vi "Configure Glitch Trigger Source.vi"(0 "VISA Resource Name":refnum<visa-resource-name>, 1 "Glitch Polarity (Positive)":i32(slide), 5 "Trigger Source (Channel 1)":string(combo)="CH1", 7 "Trigger Level (0.0 V)":dbl format="%.2p", 9 "Glitch Width (10.0e-6 s)":dbl=1e-05 format="%.2p", 11 "error in (no error)":errorcluster {"code" format="%.0x"}, 12 "Glitch Condition (Less Than)":string(combo)="Less Than") -> (4 "VISA Resource Name Out":refnum<visa-resource-name>, 15 "error out":errorcluster {"code" format="%.0x"})   [LabVIEW 2010, in "Tektronix TDS 3000 Series.lvlib"]
doc: "This VI configures the glitch trigger. A glitch trigger occurs when the trigger signal has a pulse with a width that is less than the glitch width. You specify the glitch width in the Glitch Width control. You specify the polarity of the pulse with the Glitch Polarity control. The trigger does not actually occur until the edge of a pulse that corresponds to the Glitch Width and Glitch Polarity crosses the threshold you specify in the Trigger Level control. \n\nNotes:\n\n(1) This VI affects instrument behavior only if the Trigger Type is Glitch Trigger. Call the Configure Trigger VI to set the Trigger Type before you call this VI."
uses:
  <instrlib>/Tektronix TDS 3000 Series/Tektronix TDS 3000 Series.lvlib
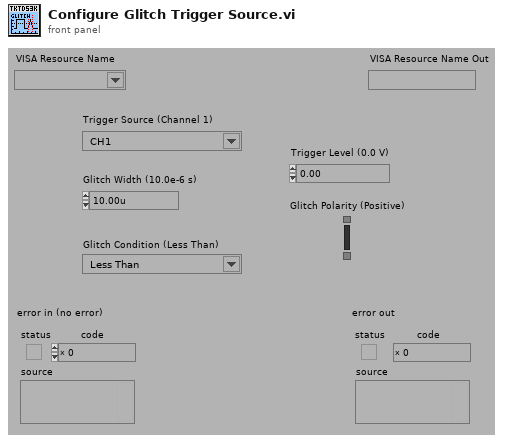
[diagram p1: front panel]
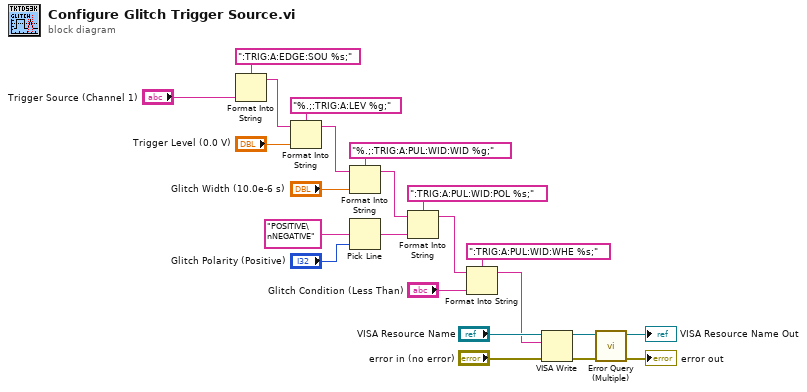
[diagram p0: block diagram]
diagram:
  n1 = Format Into String(format string=":TRIG:A:EDGE:SOU %s;", "Trigger Source (Channel 1)") -> (resulting string=w6:string)  [unwired: 2 in, 1 out]
  n2 = Format Into String(format string="%.;:TRIG:A:LEV %g;", initial string=w6, "Trigger Level (0.0 V)") -> (resulting string=w7:string)  [unwired: 1 in, 1 out]
  n3 = Format Into String(format string="%.;:TRIG:A:PUL:WID:WID %g;", initial string=w7, "Glitch Width (10.0e-6 s)") -> (resulting string=w8:string)  [unwired: 1 in, 1 out]
  n4 = Pick Line(multi-line string="POSITIVE\nNEGATIVE", line index="Glitch Polarity (Positive)") -> (output string=w13:string)  [unwired: 1 in]
  n5 = Format Into String(format string=":TRIG:A:PUL:WID:POL %s;", initial string=w8, w13) -> (resulting string=w9:string)  [unwired: 1 in, 1 out]
  n6 = Format Into String(format string=":TRIG:A:PUL:WID:WHE %s;", initial string=w9, "Glitch Condition (Less Than)") -> (resulting string=w5:string)  [unwired: 1 in, 1 out]
  n7 = VISA Write(VISA resource name="VISA Resource Name", write buffer=w5, error in (no error)="error in (no error)") -> (VISA resource name out=w4:refnum<visa-resource-name>, error out=w3:errorcluster)  [unwired: 1 out]
  n8 = call <instrlib>:"Error Query (Multiple).vi"("error in (no error)"=w3, "VISA Resource Name"=w4) -> ("error out"=→"error out":errorcluster, "VISA Resource Name Out"=→"VISA Resource Name Out":refnum<visa-resource-name>)  [unwired: 6 in, 2 out]
